vi "Point to Point VI.vi"(6 "Measurement Type":string, 7 "CalibratedImage In":T2(plugin-control), 8 "error in (no error)":errorcluster, 9 "Transformed ROI cluster":T4 {"ROI Ref [ After Transformation]"."Contours"."Type" items=["No Selection", "Point", "Line", "Rectangle", "Oval", "Polygon", "Freehand Region", "Annulus", "Unused2", "Unused3", "Broken Line", "Freehand Line", "Rotated Rectangle"]; "Measurement ROI 1 [After Transformation]"."Contours"."Type" items=["No Selection", "Point", "Line", "Rectangle", "Oval", "Polygon", "Freehand Region", "Annulus", "Unused2", "Unused3", "Broken Line", "Freehand Line", "Rotated Rectangle"]; "Measurement ROI 2 [After Transformation]"."Contours"."Type" items=["No Selection", "Point", "Line", "Rectangle", "Oval", "Polygon", "Freehand Region", "Annulus", "Unused2", "Unused3", "Broken Line", "Freehand Line", "Rotated Rectangle"]}, 10 "Measurement JSON Data":T9 {"Ref ROI Cluster"."Edge Options ROI Ref"."Edge Polarity" items=["All Edges", "Rising Edges", "Falling Edges"]; "Ref ROI Cluster"."Edge Options ROI Ref"."Minimum Edge Strength" format="%.2f"; "Ref ROI Cluster"."Edge Options ROI Ref"."Width" step=2; "Ref ROI Cluster"."Edge Options ROI Ref"."Kernel Size" step=2; "Ref ROI Cluster"."Line Options ROI Ref"."Min. Points (%)" min=0.0 max=100.0; "Ref ROI Cluster"."Line Options ROI Ref"."Min. SNR (db)" min=0.0; "Ref ROI Cluster"."Line Options ROI Ref"."Max. Score" min=0.0 max=1024.0; "Ref ROI Cluster"."Line Options ROI Ref"."Min. Score" min=0.0 max=1024.0 step=1.0; "Measurement ROI 1 Cluster"."Meas ROI 1"."Contours"."Type" items=["No Selection", "Point", "Line", "Rectangle", "Oval", "Polygon", "Freehand Region", "Annulus", "Unused2", "Unused3", "Broken Line", "Freehand Line", "Rotated Rectangle"]; "Measurement ROI 1 Cluster"."Edge Options ROI 1"."Edge Polarity" items=["All Edges", "Rising Edges", "Falling Edges"]; "Measurement ROI 1 Cluster"."Edge Options ROI 1"."Minimum Edge Strength" format="%.2f"; "Measurement ROI 1 Cluster"."Edge Options ROI 1"."Width" step=2; "Measurement ROI 1 Cluster"."Edge Options ROI 1"."Kernel Size" step=2; "Measurement ROI 1 Cluster"."Line Options ROI 1"."Min. Points (%)" min=0.0 max=100.0; "Measurement ROI 1 Cluster"."Line Options ROI 1"."Min. SNR (db)" min=0.0; "Measurement ROI 1 Cluster"."Line Options ROI 1"."Max. Score" min=0.0 max=1024.0; "Measurement ROI 1 Cluster"."Line Options ROI 1"."Min. Score" min=0.0 max=1024.0 step=1.0; "Measurement ROI 1 Cluster"."Circle Options ROI 1"."Edge Options"."Edge Polarity" items=["All Edges", "Rising Edges", "Falling Edges"]; "Measurement ROI 1 Cluster"."Circle Options ROI 1"."Edge Options"."Minimum Edge Strength" format="%.2f"; "Measurement ROI 1 Cluster"."Circle Options ROI 1"."Edge Options"."Width" step=2; "Measurement ROI 1 Cluster"."Circle Options ROI 1"."Edge Options"."Kernel Size" step=2; "Measurement ROI 2 Cluster"."Meas ROI 2"."Contours"."Type" items=["No Selection", "Point", "Line", "Rectangle", "Oval", "Polygon", "Freehand Region", "Annulus", "Unused2", "Unused3", "Broken Line", "Freehand Line", "Rotated Rectangle"]; "Measurement ROI 2 Cluster"."Edge Options ROI 2"."Edge Polarity" items=["All Edges", "Rising Edges", "Falling Edges"]; "Measurement ROI 2 Cluster"."Edge Options ROI 2"."Minimum Edge Strength" format="%.2f"; "Measurement ROI 2 Cluster"."Edge Options ROI 2"."Width" step=2; "Measurement ROI 2 Cluster"."Edge Options ROI 2"."Kernel Size" step=2; "Measurement ROI 2 Cluster"."Line Options ROI 2"."Min. Points (%)" min=0.0 max=100.0; "Measurement ROI 2 Cluster"."Line Options ROI 2"."Min. SNR (db)" min=0.0; "Measurement ROI 2 Cluster"."Line Options ROI 2"."Max. Score" min=0.0 max=1024.0; "Measurement ROI 2 Cluster"."Line Options ROI 2"."Min. Score" min=0.0 max=1024.0 step=1.0; "Measurement ROI 2 Cluster"."Circle Options ROI 2"."Edge Options"."Edge Polarity" items=["All Edges", "Rising Edges", "Falling Edges"]; "Measurement ROI 2 Cluster"."Circle Options ROI 2"."Edge Options"."Minimum Edge Strength" format="%.2f"; "Measurement ROI 2 Cluster"."Circle Options ROI 2"."Edge Options"."Width" step=2; "Measurement ROI 2 Cluster"."Circle Options ROI 2"."Edge Options"."Kernel Size" step=2}, 11 "Image In":T2(plugin-control)) -> (0 "error out":errorcluster, 2 "Measurement Value":sgl, 3 "Overlay Arrow Lines":T1)   [LabVIEW 2019, in "Algorithm.lvclass"]
uses:
  FrameworkOverrides/Algorithm.lvclass
  <vilib>/vision/NI_Vision_Development_Module.lvlib
  <vilib>/vision/Measure.llb/Edge Polarity.ctl
  <vilib>/vision/Measure.llb/Edge Options.ctl
  <vilib>/vision/Measure.llb/Straight Edge Process.ctl
  <vilib>/vision/Measure.llb/Straight Edge Options.ctl
panel:
  out "Distance":dbl format="%.2f"
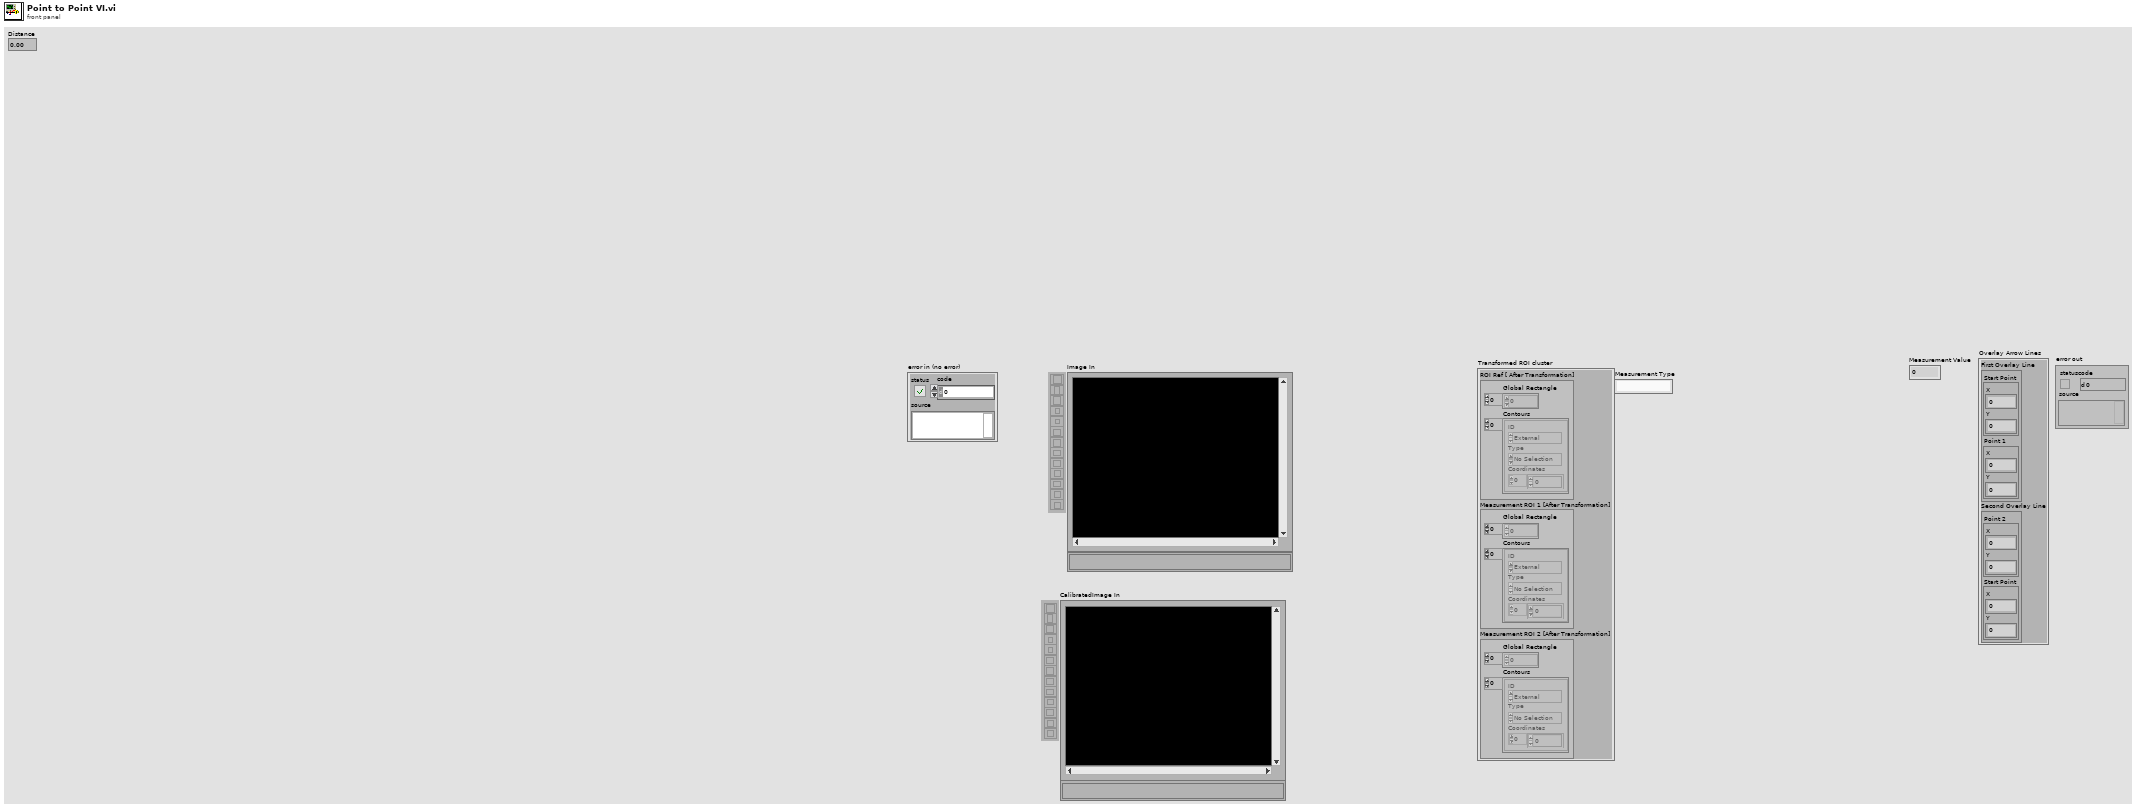
[diagram p1: front panel]
types:
  T1 = cluster{"First Overlay Line ":cluster{"Start Point":cluster{"X":sgl, "Y":sgl}, "Point 1":cluster{"X":sgl, "Y":sgl}}, "Second Overlay Line ":cluster{"Point 2":cluster{"X":sgl, "Y":sgl}, "Start Point":cluster{"X":sgl, "Y":sgl}}}
  T2 = typedef "IMAQ Image.ctl" = refnum<image>
  T3 = typedef "ROI Descriptor" = cluster{"Global Rectangle":i32[], "Contours":cluster{"ID":enum32{"External", "Internal"}, "Type":u32, "Coordinates":i32[]}[]}
  T4 = cluster{"ROI Ref [ After Transformation]":T3, "Measurement ROI 1 [After Transformation]":T3, "Measurement ROI 2 [After Transformation]":T3}
  T5 = typedef "Edge Options.ctl" = cluster{"Edge Polarity":T6, "Kernel Size":u32, "Width":u32, "Minimum Edge Strength":sgl, "Interpolation Type":enum32{"Zero Order", "Bilinear", "Quadratic", "Cubic", "Bilinear Fixed"}, "Data Processing Method":enum32{"Average", "Median"}}
  T6 = typedef "Edge Polarity.ctl" = u32
  T7 = typedef "Straight Edge Options.ctl" = cluster{"Number of Lines":i32, "Type":T8, "Min. Score":dbl, "Max. Score":dbl, "Orientation":dbl, "Angle Range":dbl, "Angle Tolerance":dbl, "Step Size":u32, "Min. SNR (db)":dbl, "Min. Points (%)":dbl, "Hough Iterations":i32}
  T8 = typedef "Straight Edge Process.ctl" = enum32{"First Edge Rake", "Best Edge Rake", "Hough Edge Rake", "First Edge Projection", "Best Edge Projection"}
  T9 = cluster{"RackID":i32, "ImageID":i32, "CameraID":i32, "MeasurementID":i32, "Measurement Name":string, "Algo Name":string, "Algo Type":string, "Ref ROI Cluster":cluster{"ROI Ref":cluster{"Global Rectangle":i32[], "Contours":cluster{"ID":enum32{"External", "Internal"}, "Type":u32, "Coordinates":i32[]}[]}, "Edge Options ROI Ref":T5, "Line Options ROI Ref":T7, "Search Direction ROI Ref":u32, "RefROIEnable":bool}, "Measurement ROI 1 Cluster":cluster{"Meas ROI 1":T3, "Edge Options ROI 1":T5, "Line Options ROI 1":T7, "Scan/Search Direction ROI 1":u16, "Step Size ROI 1":u32, "Process ROI 1":enum16{"Get First Edge", "Get First + Last Edge", "Get All Edges", "Get Best Edge"}, "Circle Options ROI 1":cluster{"Search  Direction":u32, "Edge Options":T5, "Show Search Area":bool, "Show Search Lines":bool, "Show Edges Found":bool, "Show Result":bool, "Search Area Color":u32, "Search Lines Color":u32, "Edge Locations Color":u32, "Result Color":u32, "Overlay Group Name":string}, "Circle Fit Options ROI 1":cluster{"Process":enum16{"Get First Edge", "Get First + Last Edge", "Get All Edges", "Get Best Edge"}, "Step Size":dbl, "Max Pixel Radius":i32}}, "Measurement ROI 2 Cluster":cluster{"Meas ROI 2":T3, "Edge Options ROI 2":T5, "Line Options ROI 2":T7, "Scan/Search Direction ROI 2":u32, "Step Size ROI 2":u32, "Process ROI 2":enum16{"Get First Edge", "Get First + Last Edge", "Get All Edges", "Get Best Edge"}, "Circle Options ROI 2":cluster{"Search  Direction":u32, "Edge Options":T5, "Show Search Area":bool, "Show Search Lines":bool, "Show Edges Found":bool, "Show Result":bool, "Search Area Color":u32, "Search Lines Color":u32, "Edge Locations Color":u32, "Result Color":u32, "Overlay Group Name":string}, "Circle Fit Options ROI 2":cluster{"Process":enum16{"Get First Edge", "Get First + Last Edge", "Get All Edges", "Get Best Edge"}, "Step Size":dbl, "Max Pixel Radius":i32}}, "OverlayOptions":cluster{"OverlayEnable":bool, "OverlayText":string, "OverlayCoords":i32[], "OverlayAngle":i32, "OverlayTextSize":i32, "OverlayTextColor":string, "OverlayROI":bool, "OverlayRakeLine":bool, "OverlayPoints":bool}, "MathExpression":cluster{"Algorithm":string, "MathExpression":string, "ResultVariable":string}, "MathCorrectionParameters":cluster{"Radius":dbl, "CurlGap":dbl, "Thickness":dbl, "MeasurementIndices":i32[], "MathAlgoName":string, "MathAlgoFormula":string, "CorrectionForAngle":i32[], "NumericAray":i32[], "StringArray":string[]}, "ResultVariableCluster":cluster{"RVName":string, "RVSequence":string, "RVIndex":i32, "RVID":i32, "RVValue":dbl}, "CalibrationCoefficients":cluster{"A1":dbl, "A2":dbl, "A3":dbl}, cluster{"UserCalibCoefficients":cluster{"UserCorrectionLinearityCoeff":dbl, "UserCorrectionBiasCoeff":dbl}}, "SpecValues":cluster{"LCL":dbl, "UCL":dbl, "LSL":dbl, "USL":dbl, "NominalValue":dbl}}
  T10 = cluster{"Point 2":cluster{"X":sgl, "Y":sgl}, "Start Point":cluster{"X":sgl, "Y":sgl}}
  T11 = cluster{"Start Point":cluster{"X":sgl, "Y":sgl}, "Point 1":cluster{"X":sgl, "Y":sgl}}
  T12 = cluster{"Point 1":cluster{"X":sgl, "Y":sgl}, "Point 2":cluster{"X":sgl, "Y":sgl}}
  T13 = enum16{"Get First Edge", "Get First + Last Edge", "Get All Edges", "Get Best Edge"}
  T14 = cluster{"Point1 (Pixels)":cluster{"X":sgl, "Y":sgl}, "Point2 (Pixels)":cluster{"X":sgl, "Y":sgl}, "Point1 (Real-World)":cluster{"X":sgl, "Y":sgl}, "Point2 (Real-World)":cluster{"X":sgl, "Y":sgl}, "Angle (Pixel)":dbl, "Angle (Real-World)":dbl, "Score":dbl, "Straightness":dbl, "Average SNR (db)":dbl, "Calibration Valid":bool}[]
  T15 = typedef "Search Line.ctl" = cluster{"Start Point":cluster{"X":sgl, "Y":sgl}, "End Point":cluster{"X":sgl, "Y":sgl}, "Edge Info":T16[], "Edge Map":dbl[], "Calibration Valid":bool}
  T16 = typedef "Edge New.ctl" = cluster{"Location (Pixel)":cluster{"X":sgl, "Y":sgl}, "Location (Real-World)":cluster{"X":sgl, "Y":sgl}, "Distance (Pixel)":dbl, "Distance (Real-World)":dbl, "Strength":dbl, "Noise":dbl, "Rising?":bool}
  T17 = cluster{"Point1 (Pixels)":cluster{"X":sgl, "Y":sgl}, "Point2 (Pixels)":cluster{"X":sgl, "Y":sgl}, "Point1 (Real-World)":cluster{"X":sgl, "Y":sgl}, "Point2 (Real-World)":cluster{"X":sgl, "Y":sgl}, "Angle (Pixel)":dbl, "Angle (Real-World)":dbl, "Score":dbl, "Straightness":dbl, "Average SNR (db)":dbl, "Calibration Valid":bool}
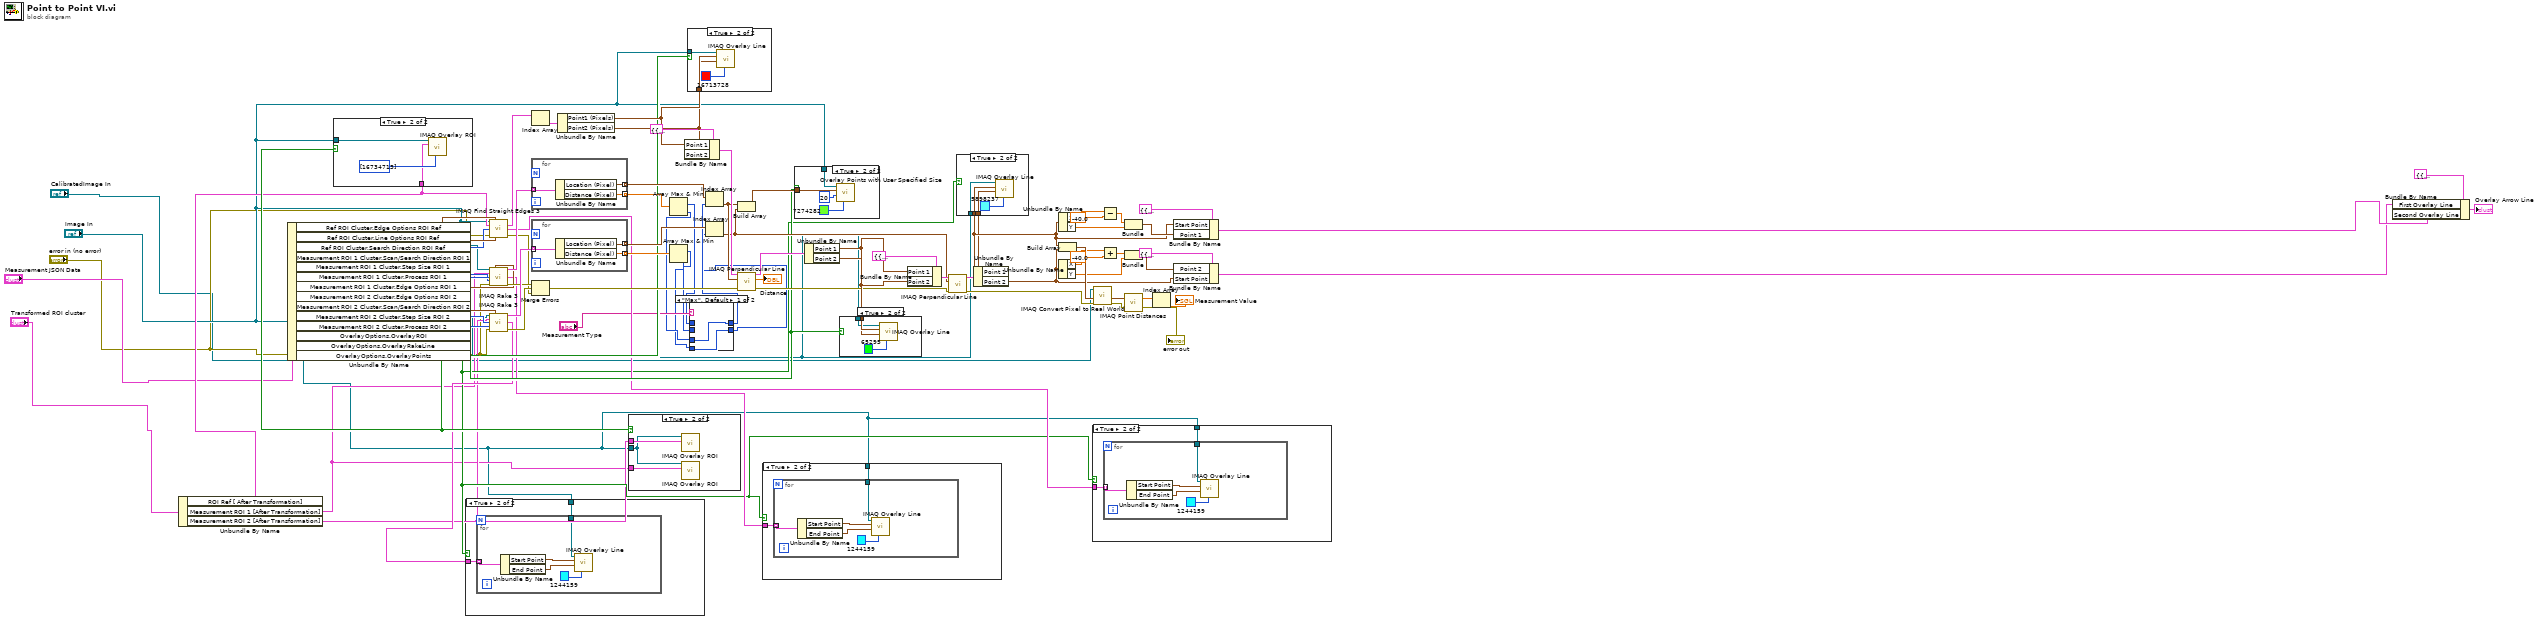
[diagram p0: block diagram]
diagram:
  n1 = Unbundle By Name("Transformed ROI cluster") -> ("ROI Ref [ After Transformation]"=w17:T3, "Measurement ROI 1 [After Transformation]"=w16:T3, "Measurement ROI 2 [After Transformation]"=w18:T3)
  n2 = Unbundle By Name("Measurement JSON Data") -> ("Ref ROI Cluster.Edge Options ROI Ref"=w52:T5, "Ref ROI Cluster.Line Options ROI Ref"=w51:T7, "Ref ROI Cluster.Search Direction ROI Ref"=w50:u32, "Measurement ROI 1 Cluster.Scan/Search Direction ROI 1"=w42:u16, "Measurement ROI 1 Cluster.Step Size ROI 1"=w43:u32, "Measurement ROI 1 Cluster.Process ROI 1"=w44:T13, "Measurement ROI 1 Cluster.Edge Options ROI 1"=w45:T5, "Measurement ROI 2 Cluster.Edge Options ROI 2"=w46:T5, "Measurement ROI 2 Cluster.Scan/Search Direction ROI 2"=w47:u32, "Measurement ROI 2 Cluster.Step Size ROI 2"=w48:u32, "Measurement ROI 2 Cluster.Process ROI 2"=w49:T13, "OverlayOptions.OverlayROI"=w24:bool, "OverlayOptions.OverlayRakeLine"=w19:bool, "OverlayOptions.OverlayPoints"=w23:bool)
  n3 = case shown="True" w24 {
    tunnel: "Image In" -> [_ w86]
    tunnel: w17 -> [_ w85]
    frame False {
    }
    frame True {
      n4 = call "IMAQ Overlay ROI"("Colors (Green)"=u32[] [16734713], "ROI Descriptor"=w85, "Image"=w86) -> ()  [unwired: 7 in, 2 out]
    }
  }
  n5 = call "IMAQ Find Straight Edges 3"("Image"="Image In", "Edge Options"=w52, "ROI Descriptor"=w17, "Search Direction"=w50, "error in (no error)"="error in (no error)", "Line Options"=w51) -> ("Straight Edges"=w75:T14, "Search Lines Information"=w20:T15[], "error out"=w76:errorcluster)  [unwired: 5 in, 2 out]
  n6 = call "IMAQ Rake 3"("Image"="Image In", "Edge Options"=w45, "ROI Descriptor"=w16, "Step Size"=w43, "Scan Direction"=w42, "error in (no error)"="error in (no error)", "Process"=w44) -> ("First Edges"=w84:T16[], "Search Lines"=w21:T15[], "error out"=w78:errorcluster)  [unwired: 5 in, 1 out]
  n7 = call "IMAQ Rake 3"("Image"="Image In", "Edge Options"=w46, "ROI Descriptor"=w18, "Step Size"=w48, "Scan Direction"=w47, "error in (no error)"="error in (no error)", "Process"=w49) -> ("First Edges"=w79:T16[], "Search Lines"=w22:T15[], "error out"=w77:errorcluster)  [unwired: 5 in, 1 out]
  n8 = case shown="True" w19 {
    tunnel: w22 -> [_ w89]
    tunnel: "Image In" -> [_ w88]
    frame False {
    }
    frame True {
      n9 = for {
        tunnel: w89 -> [w94] mode=indexing
        tunnel: w88 -> [w91]
        n10 = Unbundle By Name(w94) -> ("Start Point"=w93:cluster{"X":sgl, "Y":sgl}, "End Point"=w92:cluster{"X":sgl, "Y":sgl})
        n11 = call "IMAQ Overlay Line"("Color"=u32 1244159, "End Point"=w92, "Start Point"=w93, "Image"=w91) -> ()  [unwired: 6 in, 2 out]
      }
    }
  }
  n12 = Index Array(array=w75) -> (element=w74:T17)  [unwired: 1 in]
  n13 = for {
    tunnel: w84 -> [w97] mode=indexing
    tunnel: [w96] -> w83 mode=indexing
    tunnel: [w95] -> w82 mode=indexing
    n14 = Unbundle By Name(w97) -> ("Location (Pixel)"=w95:cluster{"X":sgl, "Y":sgl}, "Distance (Pixel)"=w96:dbl)
  }
  n15 = for {
    tunnel: w79 -> [w100] mode=indexing
    tunnel: [w99] -> w80 mode=indexing
    tunnel: [w98] -> w81 mode=indexing
    n16 = Unbundle By Name(w100) -> ("Location (Pixel)"=w98:cluster{"X":sgl, "Y":sgl}, "Distance (Pixel)"=w99:dbl)
  }
  n17 = Merge Errors(w78, w77, w76) -> (w70:errorcluster)
  n18 = Unbundle By Name(w74) -> ("Point1 (Pixels)"=w68:cluster{"X":sgl, "Y":sgl}, "Point2 (Pixels)"=w67:cluster{"X":sgl, "Y":sgl})
  n19 = case shown="True" w24 {
    tunnel: "Image In" -> [_ w101]
    tunnel: w18 -> [_ w103]
    tunnel: w16 -> [_ w102]
    frame False {
    }
    frame True {
      n20 = call "IMAQ Overlay ROI"("ROI Descriptor"=w103, "Image"=w101) -> ()  [unwired: 8 in, 2 out]
      n21 = call "IMAQ Overlay ROI"("ROI Descriptor"=w102, "Image"=w101) -> ()  [unwired: 8 in, 2 out]
    }
  }
  n22 = Array Max & Min(array=w83) -> (max index (indices)=w6:i32, min index (indices)=w2:i32)  [unwired: 2 out]
  n23 = Array Max & Min(array=w80) -> (max index (indices)=w4:i32, min index (indices)=w1:i32)  [unwired: 2 out]
  n24 = Bundle By Name(cluster=T12 {"Point 1"={"X"=0.0, "Y"=0.0}, "Point 2"={"X"=0.0, "Y"=0.0}} ("Line"), "Point 1"=w68, "Point 2"=w67) -> (w71:T12)
  n25 = case shown="True" w23 {
    tunnel: w68 -> [_ w106]
    tunnel: w67 -> [_ w105]
    tunnel: "Image In" -> [_ w104]
    frame False {
    }
    frame True {
      n26 = call "IMAQ Overlay Line"("Color"=u32 16713728, "End Point"=w105, "Start Point"=w106, "Image"=w104) -> ()  [unwired: 6 in, 2 out]
    }
  }
  n27 = case shown="\"Max\", Default" "Measurement Type" {
    tunnel: w6 -> [_ w111]
    tunnel: [w109 w111] -> w5
    tunnel: w4 -> [_ w110]
    tunnel: [w108 w110] -> w3
    tunnel: w2 -> [w109 _]
    tunnel: w1 -> [w108 _]
    frame "Max", Default {
    }
    frame "Min" {
    }
  }
  n28 = Index Array(array=w82, index=w5) -> (element=w60:cluster{"X":sgl, "Y":sgl})
  n29 = Index Array(array=w81, index=w3) -> (element=w59:cluster{"X":sgl, "Y":sgl})
  n30 = Build Array(w60, w59) -> (w73:cluster{"X":sgl, "Y":sgl}[])
  n31 = call "IMAQ Perpendicular Line"("error in (no error)"=w70, "Point"=w60, "Line"=w71) -> ("error out"=w58:errorcluster, "Distance"=→"Distance":dbl, "Perpendicular Line"=w69:T12)  [unwired: 6 in]
  n32 = case shown="True" w19 {
    tunnel: w21 -> [_ w113]
    tunnel: "Image In" -> [_ w112]
    frame False {
    }
    frame True {
      n33 = for {
        tunnel: w113 -> [w118] mode=indexing
        tunnel: w112 -> [w115]
        n34 = Unbundle By Name(w118) -> ("Start Point"=w117:cluster{"X":sgl, "Y":sgl}, "End Point"=w116:cluster{"X":sgl, "Y":sgl})
        n35 = call "IMAQ Overlay Line"("Color"=u32 1244159, "End Point"=w116, "Start Point"=w117, "Image"=w115) -> ()  [unwired: 6 in, 2 out]
      }
    }
  }
  n36 = case shown="True" w23 {
    tunnel: w73 -> [_ w122]
    tunnel: "Image In" -> [_ w119]
    frame False {
    }
    frame True {
      n37 = call "Overlay Points with User Specified Size.vi"("Color"=u32 7274282, "Point Diameter (5)"=u32 20, "Points"=w122, "Image In"=w119) -> ()  [unwired: 6 in, 2 out]
    }
  }
  n38 = Unbundle By Name(w69) -> ("Point 1"=w64:cluster{"X":sgl, "Y":sgl}, "Point 2"=w63:cluster{"X":sgl, "Y":sgl})
  n39 = case shown="True" w23 {
    tunnel: w64 -> [_ w125]
    tunnel: w63 -> [_ w124]
    tunnel: "Image In" -> [_ w123]
    frame False {
    }
    frame True {
      n40 = call "IMAQ Overlay Line"("Color"=u32 65295, "End Point"=w124, "Start Point"=w125, "Image"=w123) -> ()  [unwired: 6 in, 2 out]
    }
  }
  n41 = Bundle By Name(cluster=T12 {"Point 1"={"X"=0.0, "Y"=0.0}, "Point 2"={"X"=0.0, "Y"=0.0}} ("Line"), "Point 1"=w64, "Point 2"=w63) -> (w62:T12)
  n42 = call "IMAQ Perpendicular Line"("error in (no error)"=w58, "Point"=w59, "Line"=w62) -> ("error out"=w56:errorcluster, "Perpendicular Line"=w61:T12)  [unwired: 6 in, 1 out]
  n43 = Unbundle By Name(w61) -> ("Point 1"=w27:cluster{"X":sgl, "Y":sgl}, "Point 2"=w25:cluster{"X":sgl, "Y":sgl})
  n44 = case shown="True" w19 {
    tunnel: w27 -> [_ w129]
    tunnel: w25 -> [_ w128]
    tunnel: "Image In" -> [_ w127]
    frame False {
    }
    frame True {
      n45 = call "IMAQ Overlay Line"("Color"=u32 5898237, "End Point"=w128, "Start Point"=w129, "Image"=w127) -> ()  [unwired: 6 in, 2 out]
    }
  }
  n46 = Unbundle By Name(w27) -> ("X"=w37:sgl, "Y"=w36:sgl)
  n47 = Build Array(w27, w25) -> (w57:cluster{"X":sgl, "Y":sgl}[])
  n48 = Unbundle By Name(w25) -> ("X"=w34:sgl, "Y"=w32:sgl)
  n49 = case shown="True" w19 {
    tunnel: w20 -> [_ w132]
    tunnel: "Image In" -> [_ w131]
    frame False {
    }
    frame True {
      n50 = for {
        tunnel: w132 -> [w137] mode=indexing
        tunnel: w131 -> [w134]
        n51 = Unbundle By Name(w137) -> ("Start Point"=w136:cluster{"X":sgl, "Y":sgl}, "End Point"=w135:cluster{"X":sgl, "Y":sgl})
        n52 = call "IMAQ Overlay Line"("Color"=u32 1244159, "End Point"=w135, "Start Point"=w136, "Image"=w134) -> ()  [unwired: 6 in, 2 out]
      }
    }
  }
  n53 = call "IMAQ Convert Pixel to Real World"("error in (no error)"=w56, "Array of Pixel Coordinates"=w57, "Calibrated Image"="CalibratedImage In") -> ("error out"=w53:errorcluster, "Array of Real World Coordinates"=w55:cluster{"X":sgl, "Y":sgl}[])  [unwired: 3 in, 4 out]
  n54 = Subtract(x=w37, y=-40.0) -> (x-y=w35:dbl)
  n55 = Add(x=w34, y=-40.0) -> (x+y=w31:dbl)
  n56 = Bundle(w35, "Y"=w36) -> (w28:cluster{dbl, "Y":sgl})  [unwired: 1 in]
  n57 = Bundle(w31, "Y"=w32) -> (w26:cluster{dbl, "Y":sgl})  [unwired: 1 in]
  n58 = call "IMAQ Point Distances"("Points"=w55, "error in (no error)"=w53) -> ("Distances"=w54:sgl[], "error out"=→"error out":errorcluster)  [unwired: 3 in]
  n59 = Index Array(array=w54) -> (element=→"Measurement Value":sgl)  [unwired: 1 in]
  n60 = Bundle By Name(cluster=T11 {"Start Point"={"X"=0.0, "Y"=0.0}, "Point 1"={"X"=0.0, "Y"=0.0}} ("First Overlay Line"), "Start Point"=w27, "Point 1"=w28) -> (w30:T11)
  n61 = Bundle By Name(cluster=T10 {"Point 2"={"X"=0.0, "Y"=0.0}, "Start Point"={"X"=0.0, "Y"=0.0}} ("Second Overlay Line"), "Point 2"=w26, "Start Point"=w25) -> (w29:T10)
  n62 = Bundle By Name(cluster=T1 {"First Overlay Line "={"Start Point"={"X"=0.0, "Y"=0.0}, "Point 1"={"X"=0.0, "Y"=0.0}}, "Second Overlay Line "={"Point 2"={"X"=0.0, "Y"=0.0}, "Start Point"={"X"=0.0, "Y"=0.0}}} ("Arrow Overlay lines"), "First Overlay Line"=w29, "Second Overlay Line"=w30) -> (→"Overlay Arrow Lines":T1)
